vi "wait.vi"(7 "error in (no error)":errorcluster, 8 "ms to wait":u32) -> (1 "error out (no error)":errorcluster)   [LabVIEW 2012]
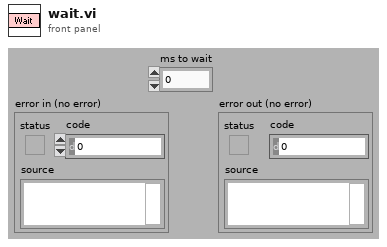
[diagram p1: front panel]
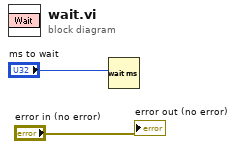
[diagram p0: block diagram]
diagram:
  n1 = Wait (ms)(milliseconds to wait="ms to wait") -> ()  [unwired: 1 out]
  "error out (no error)" <- "error in (no error)"
